vi "Analog Output - 1 Channel - N Samples.vi"() -> ()   [LabVIEW 2019]
uses:
  <vilib>/myRIO/Instrument Drivers/Onboard IO/AO Block/typedefs/AO Block Reference.ctl
  <vilib>/myRIO/Common/Instrument Driver Framework/Utilities/typedefs/myRIO Generic Hardware Reference.ctl
  <vilib>/myRIO/Common/Instrument Driver Framework/Utilities/typedefs/Hardware Version Enum.ctl
  <vilib>/myRIO/Common/Instrument Driver Framework/Utilities/typedefs/myRIO v1.0 Reference.ctl
  <vilib>/myRIO/Common/Instrument Driver Framework/Utilities/typedefs/Generic FPGA Reference.ctl
  <vilib>/myRIO/Common/Instrument Driver Framework/myRIO v1.0/AO Block/typedefs/AO Block Channels List.ctl
  <vilib>/myRIO/Common/Instrument Driver Framework/myRIO v1.0/AO Block/typedefs/AO Block Channels Enum.ctl
  <vilib>/myRIO/Common/Instrument Driver Framework/Utilities/typedefs/Analog Scaling Constants.ctl
  <vilib>/userdefined/High Color/nirio_resource_hc.ctl
  <vilib>/myRIO/Common/Instrument Driver Framework/Utilities/vis/Is FPGA Ref Available.vi
  <vilib>/myRIO/Common/Instrument Driver Framework/ELVIS III v1.0/AO Block/vis/ELVIS III v1.1 Open AO (N Samples).vi
  <vilib>/myRIO/Instrument Drivers/Onboard IO/AO Block/vis/Write.vi
  <vilib>/myRIO/Common/Instrument Driver Framework/Utilities/vis/Validate Channels.vi
  <vilib>/myRIO/Common/Instrument Driver Framework/ELVIS III v1.0/Resource Manager/vis/ELVIS III v1.0 Check For Different Banks.vi
  <vilib>/myRIO/Common/Instrument Driver Framework/myRIO v1.0/UART/vis/myRIO v1.0 Close UART.vi
  <vilib>/Utility/VariantDataType/GetNumericInfo.vi
  <vilib>/Utility/error.llb/Error Cluster From Error Code.vi
  <vilib>/myRIO/Common/Instrument Driver Framework/ELVIS III v1.0/ELVIS III v1.1 Open.vi
  <vilib>/myRIO/Common/Instrument Driver Framework/ELVIS III v1.0/AO Block/vis/ELVIS III v1.0 Reserve AO Block.vi
  <vilib>/myRIO/Common/Instrument Driver Framework/ELVIS III v1.0/Resource Manager/vis/ELVIS III v1.0 Configure DMAs.vi
  <vilib>/myRIO/Common/Instrument Driver Framework/ELVIS III v1.0/Resource Manager/vis/ELVIS III v1.0 Open Writing DMA.vi
  <vilib>/myRIO/Common/Instrument Driver Framework/myRIO v1.0/myRIO v1.0 Close.vi
  <vilib>/myRIO/Common/Instrument Driver Framework/ELVIS III v1.0/AO Block/vis/ELVIS III v1.0 AO Block Write.vi
  <vilib>/myRIO/Common/Instrument Driver Framework/Utilities/vis/FPGA Ref Manager.vi
  <vilib>/myRIO/Common/Instrument Driver Framework/ELVIS III v1.0/ELVIS III v1.0 Reset FPGA.vi
  <vilib>/myRIO/Common/Instrument Driver Framework/myRIO v1.0/IRQ/vis/myRIO v1.0 IRQ Info FGV.vi
  <vilib>/myRIO/Common/Instrument Driver Framework/myRIO v1.0/IRQ/vis/myRIO v1.0 Timer IRQ Info FGV.vi
  <vilib>/myRIO/Common/Instrument Driver Framework/myRIO v1.0/IRQ/vis/myRIO v1.0 ISR Agent.vi
  <vilib>/myRIO/Instrument Drivers/Utilities/vis/Reset Index.vi
  <vilib>/myRIO/Common/Instrument Driver Framework/myRIO v1.0/Resource Manager/vis/myRIO v1.0 Block Write Resource Manager.vi
  <vilib>/myRIO/Express VI/Onboard IO/AO/AO Express VI.xnode
  <vilib>/myRIO/Instrument Drivers/Onboard IO/AO Block/vis/myRIO AO N Samples Open.xnode
  <vilib>/myRIO/Instrument Drivers/Utilities/Utilities.lvlib
  <vilib>/myRIO/Instrument Drivers/Onboard IO/AO Block/AO Block.lvlib
panel:
  in  "Generate Waveform":bool
  in  "Frequency (Hz)":dbl=10.0 format="%#_13g"
  in  "Amplitude (V)":dbl=5.0 min=-10.0 max=10.0 step=0.1 format="%#_13g"
  in  "Stop":bool
  # "ELVIS III Control IO"
  # "模拟输出单通道"
  # "Overview: Generates one period of a sine wave on Bank A, Channel AO0 (A/AO0).\nInstructions:\n1. Configure the sine wave properties below.\n2. Connect A/AO0 to the positive lead of the load, and connect AGND to the negative lead of the load. AGND is the ground reference terminal for analog output channels.\n3. Run the VI.\n4. Press Generate Waveform to output the sine wave on A/AO0."
  # "Datasheets"
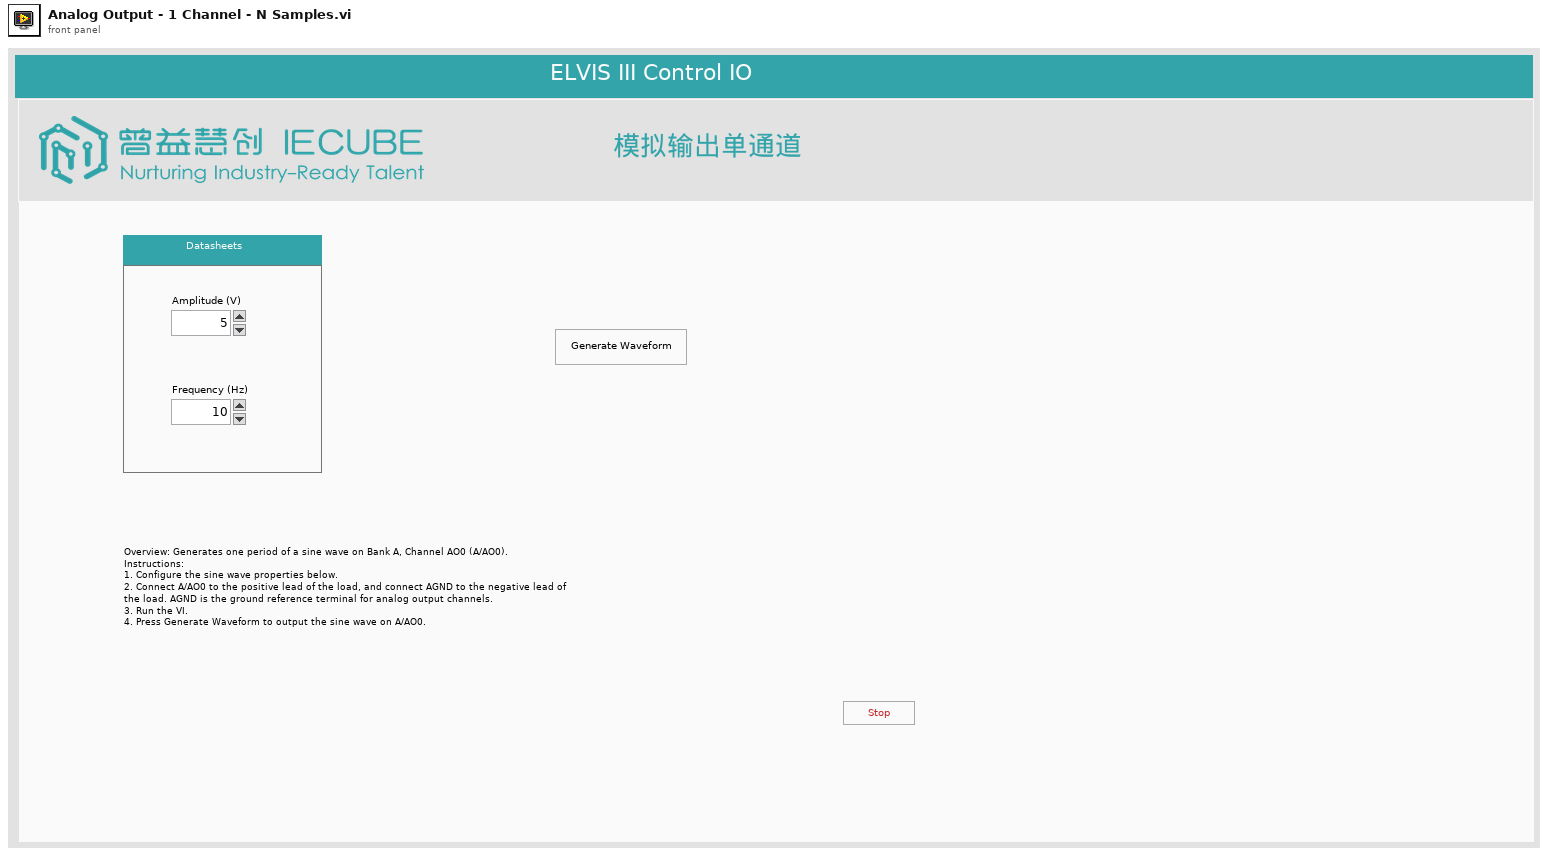
[diagram p1: front panel]
types:
  T1 = typedef "AO Block.lvlib/AO Block Reference.ctl" = cluster{"myRIO Reference":T2, "AO (N Samples) Channels List":T6, "AO (N Samples) Scaling Constants List":T8[]}
  T2 = typedef "myRIO Generic Hardware Reference.ctl" = cluster{"myRIO Model":T3, "myRIO Hardware Reference":T4}
  T3 = typedef "Hardware Version Enum.ctl" = enum16{"Unknown", "myRIO-1900", "myRIO-1950", "roboRIO", "NI ELVIS RIO CM", "ELVIS III"}
  T4 = typedef "myRIO v1.0 Reference.ctl" = cluster{"Generic FPGA Reference":T5, "Allow multiple opens":bool}
  T5 = typedef "Generic FPGA Reference.ctl" = refnum<k20>
  T6 = typedef "AO Block Channels List.ctl" = T7[]
  T7 = typedef "AO Block Channels Enum.ctl" = enum16{"Not Connected", "A/AO0 (N Samples)", "A/AO1 (N Samples)", "B/AO0 (N Samples)", "B/AO1 (N Samples)"}
  T8 = typedef "Analog Scaling Constants.ctl" = cluster{"LSB Weight (Volts)":dbl, "Offset (Volts)":dbl, "Signed?":bool}
  T9 = typedef "nirio_resource_hc.ctl" = tag
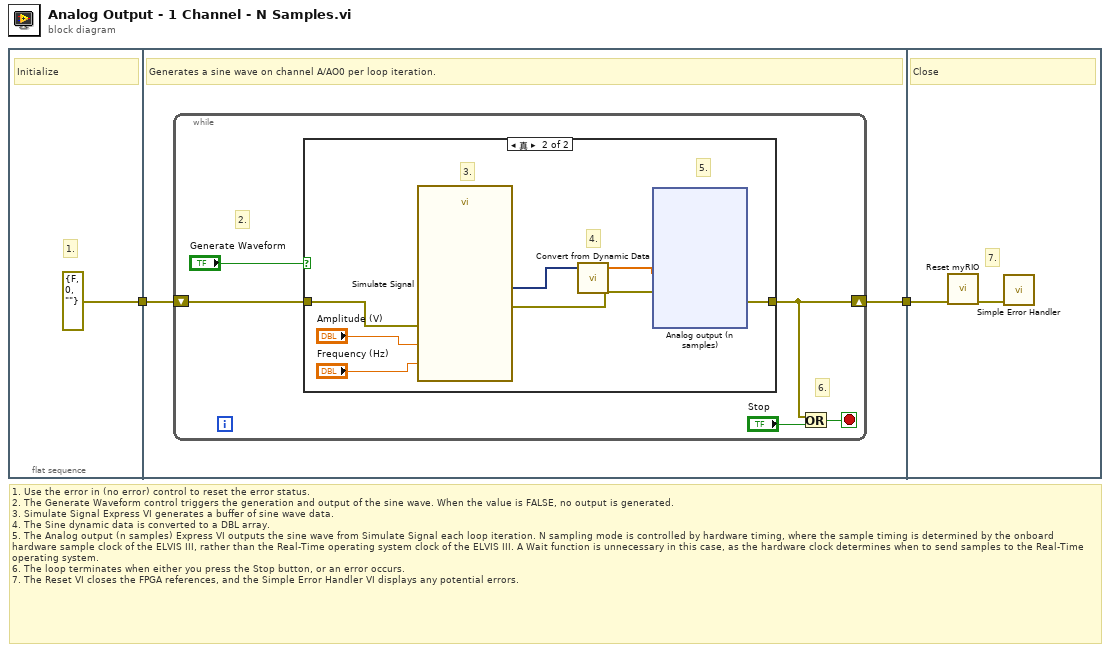
[diagram p0: block diagram]
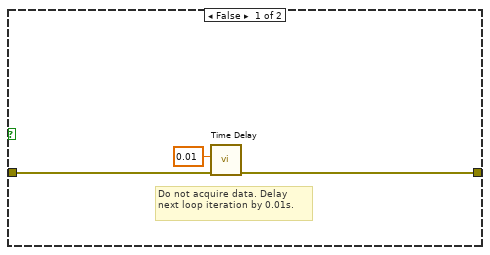
[diagram p2: hidden frame]
diagram:
  # "1. Use the error in (no error) control to reset the error status. \n2. The Generate Waveform control triggers the generation and output of the sine wave. When the value is FALSE, no output is generated.\n3. Simulate Signal Express VI generates a buffer of sine wave data.\n4. The Sine dynamic data is converted to a DBL array.\n5. The Analog output (n samples) Express VI outputs the sine wave from Simulate Signal each loop iteration. N sampling mode is controlled by hardware timing, where the sample timing is determined by the onboard hardware sample clock of the ELVIS III, rather than the Real-Time operating system clock of the ELVIS III. A Wait function is unnecessary in this case, as the hardware clock determines when to send samples to the Real-Time operating system.\n6. The loop terminates when either you press the Stop button, or an error occurs.\n7. The Reset VI closes the FPGA references, and the Simple Error Handler VI displays any potential errors."
  n1 = flat-sequence {
    tunnel: [errorcluster {"status"=FALSE, "code"=0, "source"=""} ("Error In")] -> w1
    tunnel: [w5] -> w2
    tunnel: w1 -> [w4]
    tunnel: w2 -> [w61]
    frame #0 {
      # "1."
      # "Initialize"
    }
    frame #1 {
      # "Generates a sine wave on channel A/AO0 per loop iteration."
      n2 = while {
        shift-right: [w9] -> w5
        shift-left: w4 -> [w8]
        stop <- w10 stop-if-true
        # "6."
        # "2."
        n3 = case shown="真" "Generate Waveform" {
          tunnel: [w12 w20] -> w9
          tunnel: w8 -> [w11 w19]
          frame False {
            # "Do not acquire data. Delay next loop iteration by 0.01s."
            n4 = call "Time Delay"("error in (no error)"=w11, "Delay Time (s)"=0.01) -> ("error out"=w12:errorcluster)  [unwired: 9 in]
          }
          frame True {
            # "5."
            # "4."
            # "3."
            n5 = call "Simulate Signal"("Frequency"="Frequency (Hz)", "Amplitude"="Amplitude (V)", "error in (no error)"=w19) -> ("Sine"=w15:dynamicdata, "error out"=w18:errorcluster)  [unwired: 11 in]
            n6 = call "Convert from Dynamic Data"("Dynamic Data Type"=w15) -> ("Array"=w14:dbl[])  [unwired: 3 in]
            n7 = xnode "Analog output (n samples)"("A/AO0 (N Samples)"=w14, "error in (no error)"=w18) -> ("error out"=w20:errorcluster)
          }
        }
        n8 = Or(x=w9, y="Stop") -> (x .or. y?=w10:bool)
      }
    }
    frame #2 {
      # "7."
      # "Close"
      n9 = call <vilib>:"Reset myRIO.vi"("error in (no error)"=w61) -> ("error out"=w60:errorcluster)  [unwired: 10 in]
      n10 = call <vilib>:"Simple Error Handler.vi"("error in (no error)"=w60) -> ()  [unwired: 4 in, 5 out]
    }
  }
